vi "Bytes to Bits.vi"(11 "bytes":u8[](array[numeric])) -> (3 "bits":bool[](array[boolean]))   [LabVIEW 2020, in "SubVIs.lvlib"]
doc: "This function converts an array of bytes into the equivalent number of bits."
uses:
  <vilib>/Modbus/subvis/SubVIs.lvlib
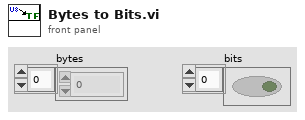
[diagram p1: front panel]
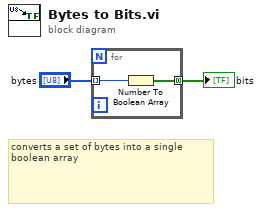
[diagram p0: block diagram]
diagram:
  # "converts a set of bytes into a single boolean array"
  n1 = for {
    tunnel: "bytes" -> [w4] mode=indexing
    tunnel: [w3] -> w1 mode=concatenating
    n2 = Number To Boolean Array(number=w4) -> (Boolean array=w3:bool[])
  }
  "bits" <- w1
